vi "Build XAPI Path.vi"(1 "SDK Directory Path":path) -> (0 "XAPI Library Path":path)   [LabVIEW 2018, in "Fujifilm X Series GFX System Digital Camera.lvlib"]
uses:
  <instrlib>/Fujifilm X Series GFX System Digital Camera/Fujifilm X Series GFX System Digital Camera.lvlib
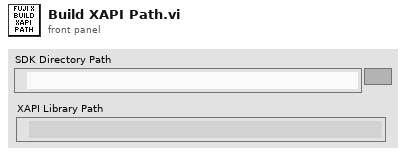
[diagram p1: front panel]
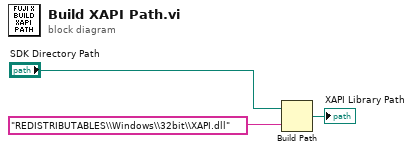
[diagram p0: block diagram]
diagram:
  n1 = Build Path(base path="SDK Directory Path", name or relative path="REDISTRIBUTABLES\\Windows\\32bit\\XAPI.dll") -> (appended path=→"XAPI Library Path":path)
